vi "TCP_server.vi"() -> ()   [LabVIEW 2018]
panel:
  in  "stop":bool
  out "receive_Data":string
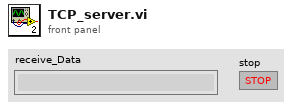
[diagram p1: front panel]
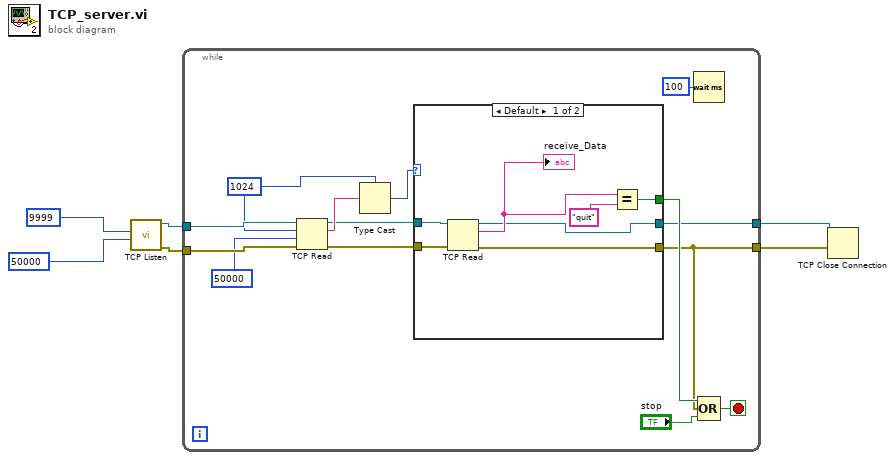
[diagram p0: block diagram]
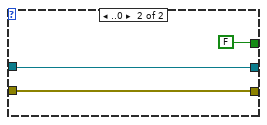
[diagram p2: hidden frame]
diagram:
  n1 = call <vilib>:"TCP Listen.vi"("timeout ms (wait forever: -1)"=50000, "port"=9999) -> ("error out"=w3:errorcluster, "connection ID"=w4:refnum<k5>)  [unwired: 5 in, 3 out]
  n2 = while {
    tunnel: w4 -> [w20]
    tunnel: w3 -> [w19]
    tunnel: [w8] -> w2
    tunnel: [w7] -> w1
    stop <- w11 stop-if-true
    w16 = 1024
    n3 = TCP Read(connection ID=w20, bytes to read=w16, error in (no error)=w19, 9:50000) -> (connection ID out=w14:refnum<k5>, data out=w17:string, error out=w13:errorcluster)  [unwired: 1 in]
    n4 = Type Cast(type=w16, x=w17) -> (*(type *) &x=w15:i32)
    n5 = case shown="Default" w15 {
      tunnel: w14 -> [w27 w30]
      tunnel: w13 -> [w26 w29]
      tunnel: [w23 FALSE] -> w9
      tunnel: [w22 w29] -> w8
      tunnel: [w21 w30] -> w7
      frame Default {
        n6 = TCP Read(connection ID=w27, error in (no error)=w26) -> (connection ID out=w21:refnum<k5>, data out=w25:string, error out=w22:errorcluster)  [unwired: 3 in]
        "receive_Data" <- w25
        n7 = Equal?(x=w25, y="quit") -> (x = y?=w23:bool)
      }
      frame ..0 {
      }
    }
    n8 = Wait (ms)(milliseconds to wait=100) -> ()  [unwired: 1 out]
    n9 = Compound Arithmetic op=OR(w9, w8, "stop") -> (w11:bool)
  }
  n10 = TCP Close Connection(connection ID=w1, error in (no error)=w2) -> ()  [unwired: 1 in, 2 out]
